vi "Create Sync Tag.vi"(7 "Blacklist":string[](array[string]), 8 "error in (no error)":errorcluster, 9 "Parent Type":T1, 11 "Variable":refnum<k21>) -> (0 "error out":errorcluster, 2 "Created?":bool, 3 "Synchronised Tag":refnum<class "Synchronised Tag.lvclass">, 4 "Folder":string)   [LabVIEW 2016, in "Synchronised Tag.lvclass"]
doc: "Takes a variable path, opens the connection and then creates a variant with all the information required later."
uses:
  Synchronised Tag.lvclass
  Controls/Node Type.ctl
  Controls/Access Mode.ctl
  Synchronised Tag.lvclass/Synchronised Tag.ctl
  <resource>/objmgr/ni.var.rc
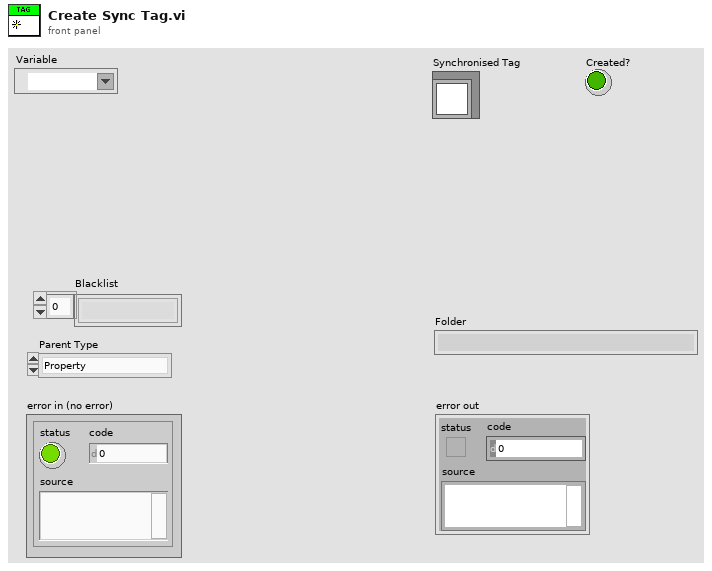
[diagram p1: front panel]
types:
  T1 = typedef "Node Type.ctl" = enum16{"Property", "Item", "Folder"}
  T2 = typedef "Synchronised Tag.lvclass/Access Mode.ctl" = enum16{"Unused", "Read Only", "Write Only", "Read/Write"}
  T3 = typedef "OPC type.ctl" = u16
  T4 = typedef "SV type.ctl" = enum16{"Boolean", "SByte", "Byte", "Int16", "UInt16", "Int32", "UInt32", "Int64", "UInt64", "Float", "Double", "String", "DateTime", "ByteString", "Array of Boolean", "Array of SByte", "Array of Byte", "Array of Int16", "Array of UInt16", "Array of Int32", "Array of UInt32", "Array of Int64", "Array of UInt64", "Array of Float", "Array of Double", "Array of String", "Array of DateTime", "Array of ByteString", "Unsupported"}
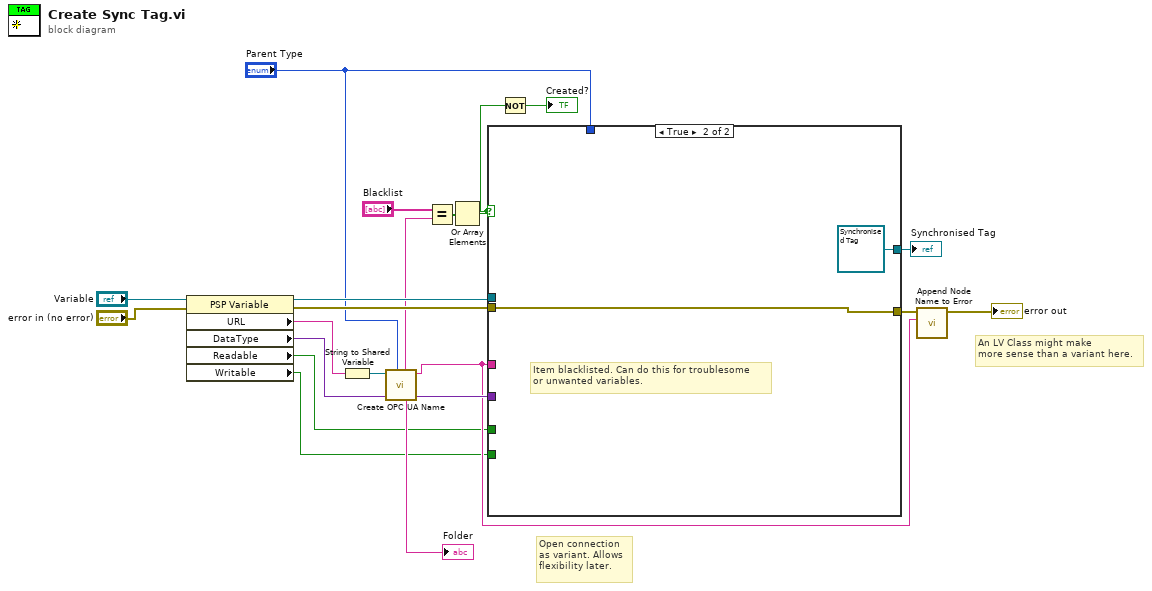
[diagram p0: block diagram]
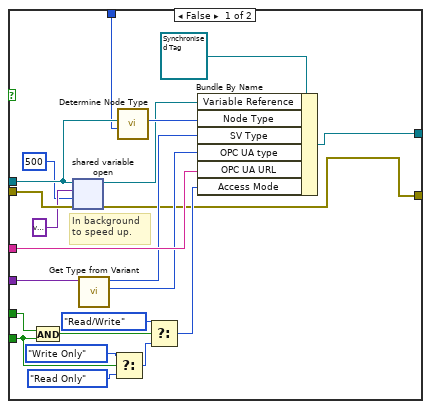
[diagram p2: hidden frame]
diagram:
  # "Open connection\nas variant. Allows\nflexibility later."
  # "An LV Class might make\nmore sense than a variant here."
  n1 = property class="PSP Variable"(reference="Variable", error in="error in (no error)") -> (reference out=w18:refnum<k21>, error out=w16:errorcluster, "URL"=w20:string, "DataType"=w17:variant, "Readable"=w2:bool, "Writable"=w3:bool)
  n2 = String to Shared Variable(0:w20) -> (2:w19:refnum<k21>)  [unwired: 1 out]
  n3 = call "Create OPC UA Name.vi"("Parent Type"="Parent Type", "SV"=w19) -> ("Path"=w6:string, "Folder"=→"Folder":string, "Name"=w10:string)  [unwired: 7 in]
  n4 = Equal?(x="Blacklist", y=w10) -> (x = y?=w13:bool[])
  n5 = Or Array Elements(Boolean array=w13) -> (logical OR=w12:bool)
  n6 = case shown="True" w12 {
    tunnel: w18 -> [w35 _]
    tunnel: w17 -> [w42 _]
    tunnel: w16 -> [w41 w44]
    tunnel: [w22 w44] -> w8
    tunnel: w6 -> [w38 _]
    tunnel: "Parent Type" -> [w34 _]
    tunnel: [w21 refnum<class "Synchronised Tag.lvclass"> refnum ("Synchronised Tag.lvclass")] -> w1
    tunnel: w3 -> [w27 _]
    tunnel: w2 -> [w30 _]
    frame False {
      # "In background\nto speed up."
      n7 = And(x=w30, y=w27) -> (x .and. y?=w29:bool)
      n8 = shared-variable-open(w35, w41, variant ("variant"), 500 ("timeout ms")) -> (w32:refnum<k21>, w22:errorcluster)  [unwired: 2 in]
      n9 = call "Get Type from Variant.vi"("Data Type"=w42) -> ("OPC UA Data Type"=w36:T3, "SV Data Type"=w37:T4)  [unwired: 9 in]
      n10 = Select(t=Access_Mode."Write Only" ("Access Mode"), s=w27, f=Access_Mode."Read Only" ("Access Mode")) -> (s? t:f=w28:T2)
      n11 = call "Determine Node Type.vi"("Parent Type"=w34, "Refnum in"=w35) -> ("Node Type"=w33:T1)  [unwired: 9 in]
      n12 = Select(t=Access_Mode."Read/Write" ("Access Mode"), s=w29, f=w28) -> (s? t:f=w23:T2)
      n13 = Bundle By Name(cluster=refnum<class "Synchronised Tag.lvclass"> refnum ("Synchronised Tag.lvclass"), "Variable Reference"=w32, "Node Type"=w33, "SV Type"=w37, "OPC UA type"=w36, "OPC UA URL"=w38, "Access Mode"=w23) -> (w21:refnum<class "Synchronised Tag.lvclass">)
    }
    frame True {
      # "Item blacklisted. Can do this for troublesome\nor unwanted variables."
    }
  }
  "Synchronised Tag" <- w1
  n14 = Not(x=w12) -> (.not. x?=→"Created?":bool)
  n15 = call "Append Node Name to Error.vi"("Node Name"=w6, "error in (no error)"=w8) -> ("error out"=→"error out":errorcluster)  [unwired: 9 in]
